vi "myRIO_BRig_RT_dataBlock_nRewards__R.vi"() -> (2 "output_nRewards__R":i32)   [LabVIEW 2014]
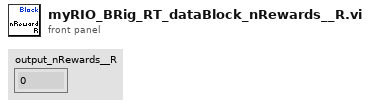
[diagram p1: front panel]
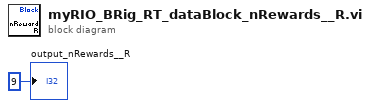
[diagram p0: block diagram]
diagram:
  "output_nRewards__R" <- 9 ("output_iBlock")
